vi "Load_Profile_Example.vi"(4 "PS VISA in":refnum<visa-resource-name>, 5 "PS error in":errorcluster, 12 "Output Safety":T1, 13 "Current Cutoff":dbl) -> (18 "PS VIS resource name out":refnum<visa-resource-name>, 19 "PS error out":errorcluster)   [LabVIEW 2020]
uses:
  <vilib>/Utility/file.llb/Read Delimited Spreadsheet (DBL).vi
  Drivers-NHR-9200/NHR/Public/Data/Low Level/Fetch (Ave Voltage).vi
  Drivers-NHR-9200/NHR/NH Research Regenerative Test Series.lvlib
panel:
  in  "ChargeCyclePath":string
  in  "DischargeCyclePath":string
  out "Read Ave Voltage (V) 2":dbl
  out "Read Ave Current (A) 2":dbl
  in  "cycles":i32
  in  "file path":path
  in  "format (%.3f)":string="%.3f"
  out "Read Ave Current (A)":dbl
  out "Read Ave Voltage (V)":dbl
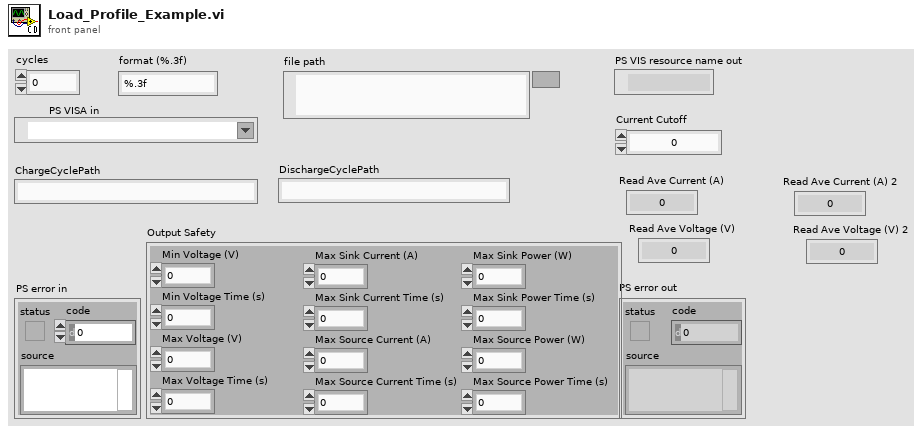
[diagram p1: front panel]
types:
  T1 = cluster{"Min Voltage (V)":dbl, "Min Voltage Time (s)":dbl, "Max Voltage (V)":dbl, "Max Voltage Time (s)":dbl, "Max Sink Current (A)":dbl, "Max Sink Current Time (s)":dbl, "Max Source Current (A)":dbl, "Max Source Current Time (s)":dbl, "Max Sink Power (W)":dbl, "Max Sink Power Time (s)":dbl, "Max Source Power (W)":dbl, "Max Source Power Time (s)":dbl}
  T2 = cluster{"Voltage Enabled":bool, "Current Enabled":bool, "Power Enabled":bool, "Resistance Enabled":bool}
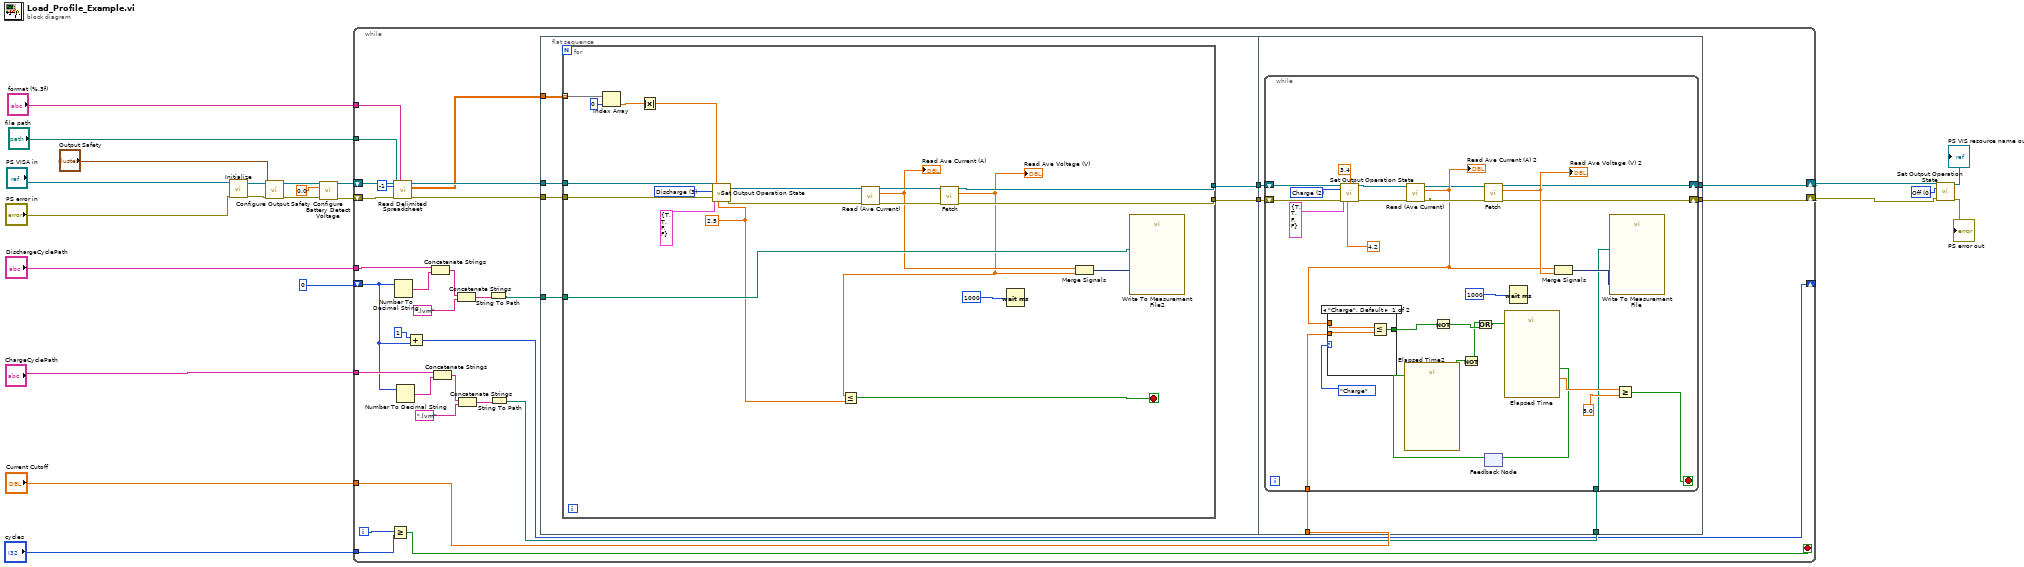
[diagram p0: block diagram]
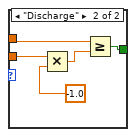
[diagram p2: hidden frame]
diagram:
  w6 = 0 items=["Off", "Standby", "Charge", "Discharge", "Battery"] ("Mode (0: Off)")
  n1 = call "Initialize.vi"("VISA resource name"="PS VISA in", "error in (no error)"="PS error in") -> ("VISA resource name out"=w17:refnum<visa-resource-name>, "error out"=w18:errorcluster)  [unwired: 12 in]
  n2 = call "Configure Output Safety.vi"("VISA resource name"=w17, "Output Safety"="Output Safety", "error in (no error)"=w18) -> ("VISA resource name out"=w20:refnum<visa-resource-name>, "error out"=w19:errorcluster)  [unwired: 11 in]
  n3 = call "Configure Battery Detect Voltage.vi"("VISA resource name"=w20, "Battery Detect Voltage (0V)"=0.0, "error in (no error)"=w19) -> ("VISA resource name out"=w13:refnum<visa-resource-name>, "error out"=w11:errorcluster)  [unwired: 11 in]
  n4 = while {
    tunnel: "Current Cutoff" -> [w40]
    tunnel: "format (%.3f)" -> [w52]
    tunnel: "file path" -> [w51]
    shift-right: [w38] -> w4
    shift-left: w13 -> [w49]
    shift-right: [w39] -> w5
    shift-left: w11 -> [w47]
    tunnel: "cycles" -> [w44]
    tunnel: "ChargeCyclePath" -> [w27]
    shift-right: [w23] -> _
    shift-left: 0 ("number of rows (all:-1)") -> [w24]
    tunnel: "DischargeCyclePath" -> [w36]
    i -> [w45]
    stop <- w43 stop-if-true
    n5 = Greater Or Equal?(x=w45, y=w44) -> (x >= y?=w43:bool)
    n6 = call-poly <vilib>:"Read Delimited Spreadsheet.vi"("file path (dialog if empty)"=w51, "format (%.3f)"=w52, "number of rows (all:-1)"=-1, "error in (no error)"=w47) -> ("all rows"=w48:dbl[][], "error out"=w46:errorcluster)  [unwired: 6 in, 4 out]
    n7 = Number To Decimal String(number=w24) -> (decimal integer string=w34:string)  [unwired: 1 in]
    n8 = Number To Decimal String(number=w24) -> (decimal integer string=w29:string)  [unwired: 1 in]
    n9 = Add(x=1 ("number of rows (all:-1)"), y=w24) -> (x+y=w23:i32)
    n10 = Concatenate Strings(w36, w34) -> (w35:string)
    n11 = Concatenate Strings(w27, w29) -> (w30:string)
    n12 = Concatenate Strings(w35, ".lvm" ("concatenated string")) -> (w33:string)
    n13 = Concatenate Strings(w30, ".lvm" ("concatenated string")) -> (w28:string)
    n14 = String To Path(string=w33) -> (path=w32:path)
    n15 = String To Path(string=w28) -> (path=w26:path)
    n16 = flat-sequence {
      tunnel: w32 -> [w53]
      tunnel: w49 -> [w58]
      tunnel: w48 -> [w57]
      tunnel: w46 -> [w56]
      tunnel: [w55] -> w42
      tunnel: [w54] -> w41
      tunnel: [w82] -> w39
      tunnel: [w83] -> w38
      tunnel: w42 -> [w85]
      tunnel: w41 -> [w84]
      tunnel: w40 -> [w81]
      tunnel: w26 -> [w80]
      frame #0 {
        n17 = for {
          tunnel: w53 -> [w75]
          tunnel: [w74] -> w55
          tunnel: [w73] -> w54
          tunnel: w58 -> [w67]
          tunnel: w56 -> [w65]
          tunnel: w57 -> [w68] mode=indexing
          stop <- w59 stop-if-true
          w69 = 2.5 ("Charge/Discharge Voltage Setpoint")
          w60 = 3 items=["Off", "Standby", "Charge", "Discharge", "Battery"] ("Mode (0: Off)")
          n18 = Index Array(array=w68, index=0 ("disabled index (row)")) -> (element=w62:dbl)
          n19 = Absolute Value(x=w62) -> (abs(x)=w66:dbl)
          n20 = call "Set Output Operation State.vi"("VISA resource name"=w67, "Voltage Setpoint (0 V)"=w69, "Current Setpoint (0 A)"=w66, "Mode (0: Off)"=w60, "Enable"=T2 {"Voltage Enabled"=TRUE, "Current Enabled"=TRUE, "Power Enabled"=FALSE, "Resistance Enabled"=FALSE}, "error in (no error)"=w65) -> ("VISA resource name out"=w64:refnum<visa-resource-name>, "error out"=w63:errorcluster)  [unwired: 8 in]
          n21 = call "Read (Ave Current).vi"("VISA resource name"=w64, "error in (no error)"=w63) -> ("VISA resource name out"=w78:refnum<visa-resource-name>, "Ave Current (A)"=w72:dbl, "error out"=w79:errorcluster)  [unwired: 11 in]
          "Read Ave Current (A)" <- w72
          n22 = call-poly "Fetch.vi"("VISA resource name"=w78, "error in (no error)"=w79) -> ("VISA resource name out"=w74:refnum<visa-resource-name>, "Ave Voltage (V)"=w71:dbl, "error out"=w73:errorcluster)  [unwired: 11 in]
          "Read Ave Voltage (V)" <- w71
          n23 = Less Or Equal?(x=w71, y=w69) -> (x <= y?=w59:bool)
          n24 = Wait (ms)(milliseconds to wait=1000) -> ()  [unwired: 1 out]
          n25 = Merge Signals "Merge Signals"(w72, w71) -> (w77:dynamicdata)
          n26 = call "Write To Measurement File2"("Signals"=w77, "Filename"=w75) -> ()  [unwired: 15 in, 3 out]
        }
      }
      frame #1 {
        n27 = while {
          shift-right: [w93] -> w83
          shift-left: w85 -> [w110]
          shift-right: [w92] -> w82
          shift-left: w84 -> [w109]
          tunnel: w81 -> [w98]
          tunnel: w80 -> [w91]
          stop <- w99 stop-if-true
          w112 = 4.2 ("Charge/Discharge Voltage Setpoint")
          w114 = 2 items=["Off", "Standby", "Charge", "Discharge", "Battery"] ("Mode (0: Off)")
          n28 = call "Set Output Operation State.vi"("VISA resource name"=w110, "Voltage Setpoint (0 V)"=w112, "Current Setpoint (0 A)"=3.4 ("Voltage Setpoint (0 V)"), "Mode (0: Off)"=w114, "Enable"=T2 {"Voltage Enabled"=TRUE, "Current Enabled"=TRUE, "Power Enabled"=FALSE, "Resistance Enabled"=FALSE}, "error in (no error)"=w109, "Power Setpoint (0 W)"=w112) -> ("VISA resource name out"=w86:refnum<visa-resource-name>, "error out"=w90:errorcluster)  [unwired: 7 in]
          n29 = call "Read (Ave Current).vi"("VISA resource name"=w86, "error in (no error)"=w90) -> ("VISA resource name out"=w87:refnum<visa-resource-name>, "Ave Current (A)"=w88:dbl, "error out"=w89:errorcluster)  [unwired: 11 in]
          "Read Ave Current (A) 2" <- w88
          n30 = case shown="\"Charge\", Default" enum8{"Charge", "Discharge"}."Charge" ("Charge/discharge 2") {
            tunnel: w98 -> [w116 w121]
            tunnel: w88 -> [w117 w119]
            tunnel: [w115 w118] -> w100
            frame "Charge", Default {
              n31 = Less Or Equal?(x=w117, y=w116) -> (x <= y?=w115:bool)
            }
            frame "Discharge" {
              n32 = Multiply(x=w121, y=-1.0) -> (x*y=w120:dbl)
              n33 = Greater Or Equal?(x=w119, y=w120) -> (x >= y?=w118:bool)
            }
          }
          n34 = Not(x=w100) -> (.not. x?=w108:bool)
          n35 = call-poly "Fetch.vi"("VISA resource name"=w87, "error in (no error)"=w89) -> ("VISA resource name out"=w93:refnum<visa-resource-name>, "Ave Voltage (V)"=w95:dbl, "error out"=w92:errorcluster)  [unwired: 11 in]
          "Read Ave Voltage (V) 2" <- w95
          n36 = feedback #1() -> (w101:bool)  [unwired: 1 in]
          n37 = call "Elapsed Time2"("Reset"=w101) -> ("Time has Elapsed"=w107:bool)  [unwired: 11 in, 7 out]
          n38 = Not(x=w107) -> (.not. x?=w106:bool)
          n39 = Or(x=w106, y=w108) -> (x .or. y?=w105:bool)
          n40 = call "Elapsed Time"("Reset"=w105) -> ("Elapsed Time (s)"=w104:dbl, "Time has Elapsed"=w102:bool)  [unwired: 11 in, 6 out]
          n41 = feedback-in #1(w102) -> ()
          n42 = Wait (ms)(milliseconds to wait=1000) -> ()  [unwired: 1 out]
          n43 = Merge Signals "Merge Signals"(w88, w95) -> (w97:dynamicdata)
          n44 = call "Write To Measurement File"("Signals"=w97, "Filename"=w91) -> ()  [unwired: 15 in, 3 out]
          n45 = Greater Or Equal?(x=w104, y=5.0) -> (x >= y?=w99:bool)
        }
      }
    }
  }
  n46 = call "Set Output Operation State.vi"("VISA resource name"=w4, "Mode (0: Off)"=w6, "error in (no error)"=w5) -> ("VISA resource name out"=→"PS VIS resource name out":refnum<visa-resource-name>, "error out"=→"PS error out":errorcluster)  [unwired: 11 in]
